vi "Complete Measurament RT.vi"() -> ()   [LabVIEW 2014]
uses:
  <vilib>/Platform/TimedLoop/XDataNode/timing_clust.ctl
  <vilib>/Platform/TimedLoop/XDataNode/nitl_modes.ctl
  <vilib>/Platform/TimedLoop/XDataNode/wakeup.ctl
  <vilib>/Analysis/3filter.llb/Filter Passband Type.ctl
  <vilib>/Analysis/Matrix/Datatypes/RealMatrix.ctl
  <vilib>/FPGAPlugInAG/sbRIO-9636/niLvFpga_Open_sbRIO-9636.vi
  <vilib>/rvi/interface/common/dynamic/niFpgaDynamicAddResources.vi
  <vilib>/FPGAPlugInAG/Dynamic/niLvFpga_Reset_Dynamic.vi
  <vilib>/Utility/error.llb/Error Cluster From Error Code.vi
  <vilib>/rvi/errors/niLvFpgaAdjustHostInterfaceError.vi
  <vilib>/rvi/interface/common/niFpgaWaitOnOcc.vi
  <vilib>/Analysis/3filter.llb/Butterworth Filter (DBL).vi
  <vilib>/FPGAPlugInAG/Dynamic/niLvFpga_Run_Dynamic.vi
  <vilib>/FPGAPlugInAG/Dynamic/niLvFpga_Abort_Dynamic.vi
  <vilib>/FPGAPlugInAG/Dynamic/niLvFpga_Close_Dynamic.vi
  <vilib>/rvi/interface/nirviOpenFPGA/nirviOpenFPGA.xnode
  FPGA Bitfiles/LaserDistanceSen_FPGATarget_N-ParametricDoub_YVLbjAYtdP4.lvbitx
  FPGA Target/Test VIs/N-Parametric Double FFT Mesurament Test.vi
  FPGA Bitfiles/LaserDistanceSen_FPGATarget_N-ParametricDoub_qx5IM88U9d4.lvbitx
  FPGA Target/Test VIs/N-Parametric Double FFT Mesurament Test SLOW.vi
  <vilib>/rvi/interface/nirviMethod/nirviMethod.xnode
  <vilib>/rvi/interface/nirviReadWriteControl/nirviReadWriteControl.xnode
  <vilib>/Platform/TimedLoop/XDataNode/XDataNode.xnode
  <vilib>/rvi/interface/nirviCloseFPGA/nirviCloseFPGA.xnode
  <vilib>/FPGAPlugInAG/Dynamic/niLvFpga_ConfigureFifo_Dynamic.vi
  <vilib>/rvi/errors/niLvFpgaMergeErrorWithErrorCode.vi
  <vilib>/FPGAPlugInAG/Dynamic/niLvFpga_StartFifo_Dynamic.vi
  <vilib>/rvi/interface/Simulation/niFpgaSimulationCallBeginRW.vi
  <vilib>/FPGAPlugInAG/Dynamic/niLvFpga_ReadFifo_Dynamic.vi
  <vilib>/Platform/TimedLoop/XDataNode/XDNodeRunTimeDep.lvlib
  NiFpgaLv.dll
  <vilib>/Analysis/NI_AALBase.lvlib
  <vilib>/Analysis/Matrix/NI_Matrix.lvlib
panel:
  out "Distance ONLINE":dbl[](graph)
  in  "Low cutoff freq":dbl=200000.0 format="%#_13g"
  in  "Tri Low pass filter":bool
  in  "3 point interpolation algorithm":bool
  in  "Mov mean":bool
  out "moving mean speed":dbl format="%0.7f"
  out "moving standard deviation rel speed":dbl format="%0.7f"
  in  "#movesignal 2":i32=100
  out "moving freq mean":dbl
  in  "Tab Control":enum32{"5 bin", "5 bin mean", "Distance "}(tab)=enum."Distance "
  out "5 bin FALL":T1(graph) caption="5 freq fall"
  out "5 bin RISE":T1(graph)
  out "5 bin mean/std FALL":T2(graph)
  in  "#meanBin":i32=100
  out "5 bin mean/std RISE":T2(graph)
  out "Distance and error":T1(graph)
  out "Speed and error":T1(graph)
  in  "Lin Mes":bool
  in  "step (m)":dbl=0.0001
  out "Max peak-peak error (m)":dbl
  out "Mean error (m)":dbl
  in  "Plot":bool
  in  "Sample /Modulation Frequency":enum32{"40MHz/32KHz", "30MHz/24Khz"}(radio)=enum."30MHz/24Khz"
  in  "#movesignal":i32=100
  out "moving standard deviation rel":dbl format="%0.7f"
  out "moving mean":dbl format="%0.7f"
  out "StdDev Rel 1":dbl
  out "StdDev Rel 2":dbl
  out "Warning":bool
  out "Velocity (m/s)":dbl
  out "Distance (m)":dbl
  out "Mean Frequency":dbl
  out "Rise array size":i32
  out "Fall array size":i32
  out "Mean Frequency Rising (Hz)":dbl
  out "Mean Frequency Falling (Hz)":dbl
  in  "tieni premuto per":i32=100
  in  "Triangular Multiply Factor":dbl[](array[numeric])=[1.0, 0.8, 0.95, 0.85, 0.9]
  out "RISING Second Edge N-FFT":dbl[](graph)
  in  "Enable triangular scaling":bool=TRUE
  in  "Triangolo dritto?":bool
  out "FALLING First Edge N-FFT":dbl[](graph)
  in  "#Signals":u32(slide)=5 scale=1.0..5.0
  in  "stop":bool
  in  "Initial Latency points":u32(slide) scale=0.0..1249.0
  out "Elements Remaining FFT":u32
  out "Elements Remaining Signal":u32
  out "N-Signals":dbl[](graph)
  in  "Snapshot":bool
  in  "Windowing":T3(ring)=enum."Hanning"
  in  "first bin":i32=5
  in  "last bin":i32=255
  in  "lower limit 2":u32(slide)=738 scale=625.0..738.0
  in  "lower limit 1":u32(slide)=113 scale=0.0..113.0
  # "OFFLINE parameters"
  # "200k/400k"
  # "Max Detection FFT bin range"
  # "WARNING:\nOnce pressed wait untill the end of operation"
  # "Distance"
  # "Mean"
  # "Velocity"
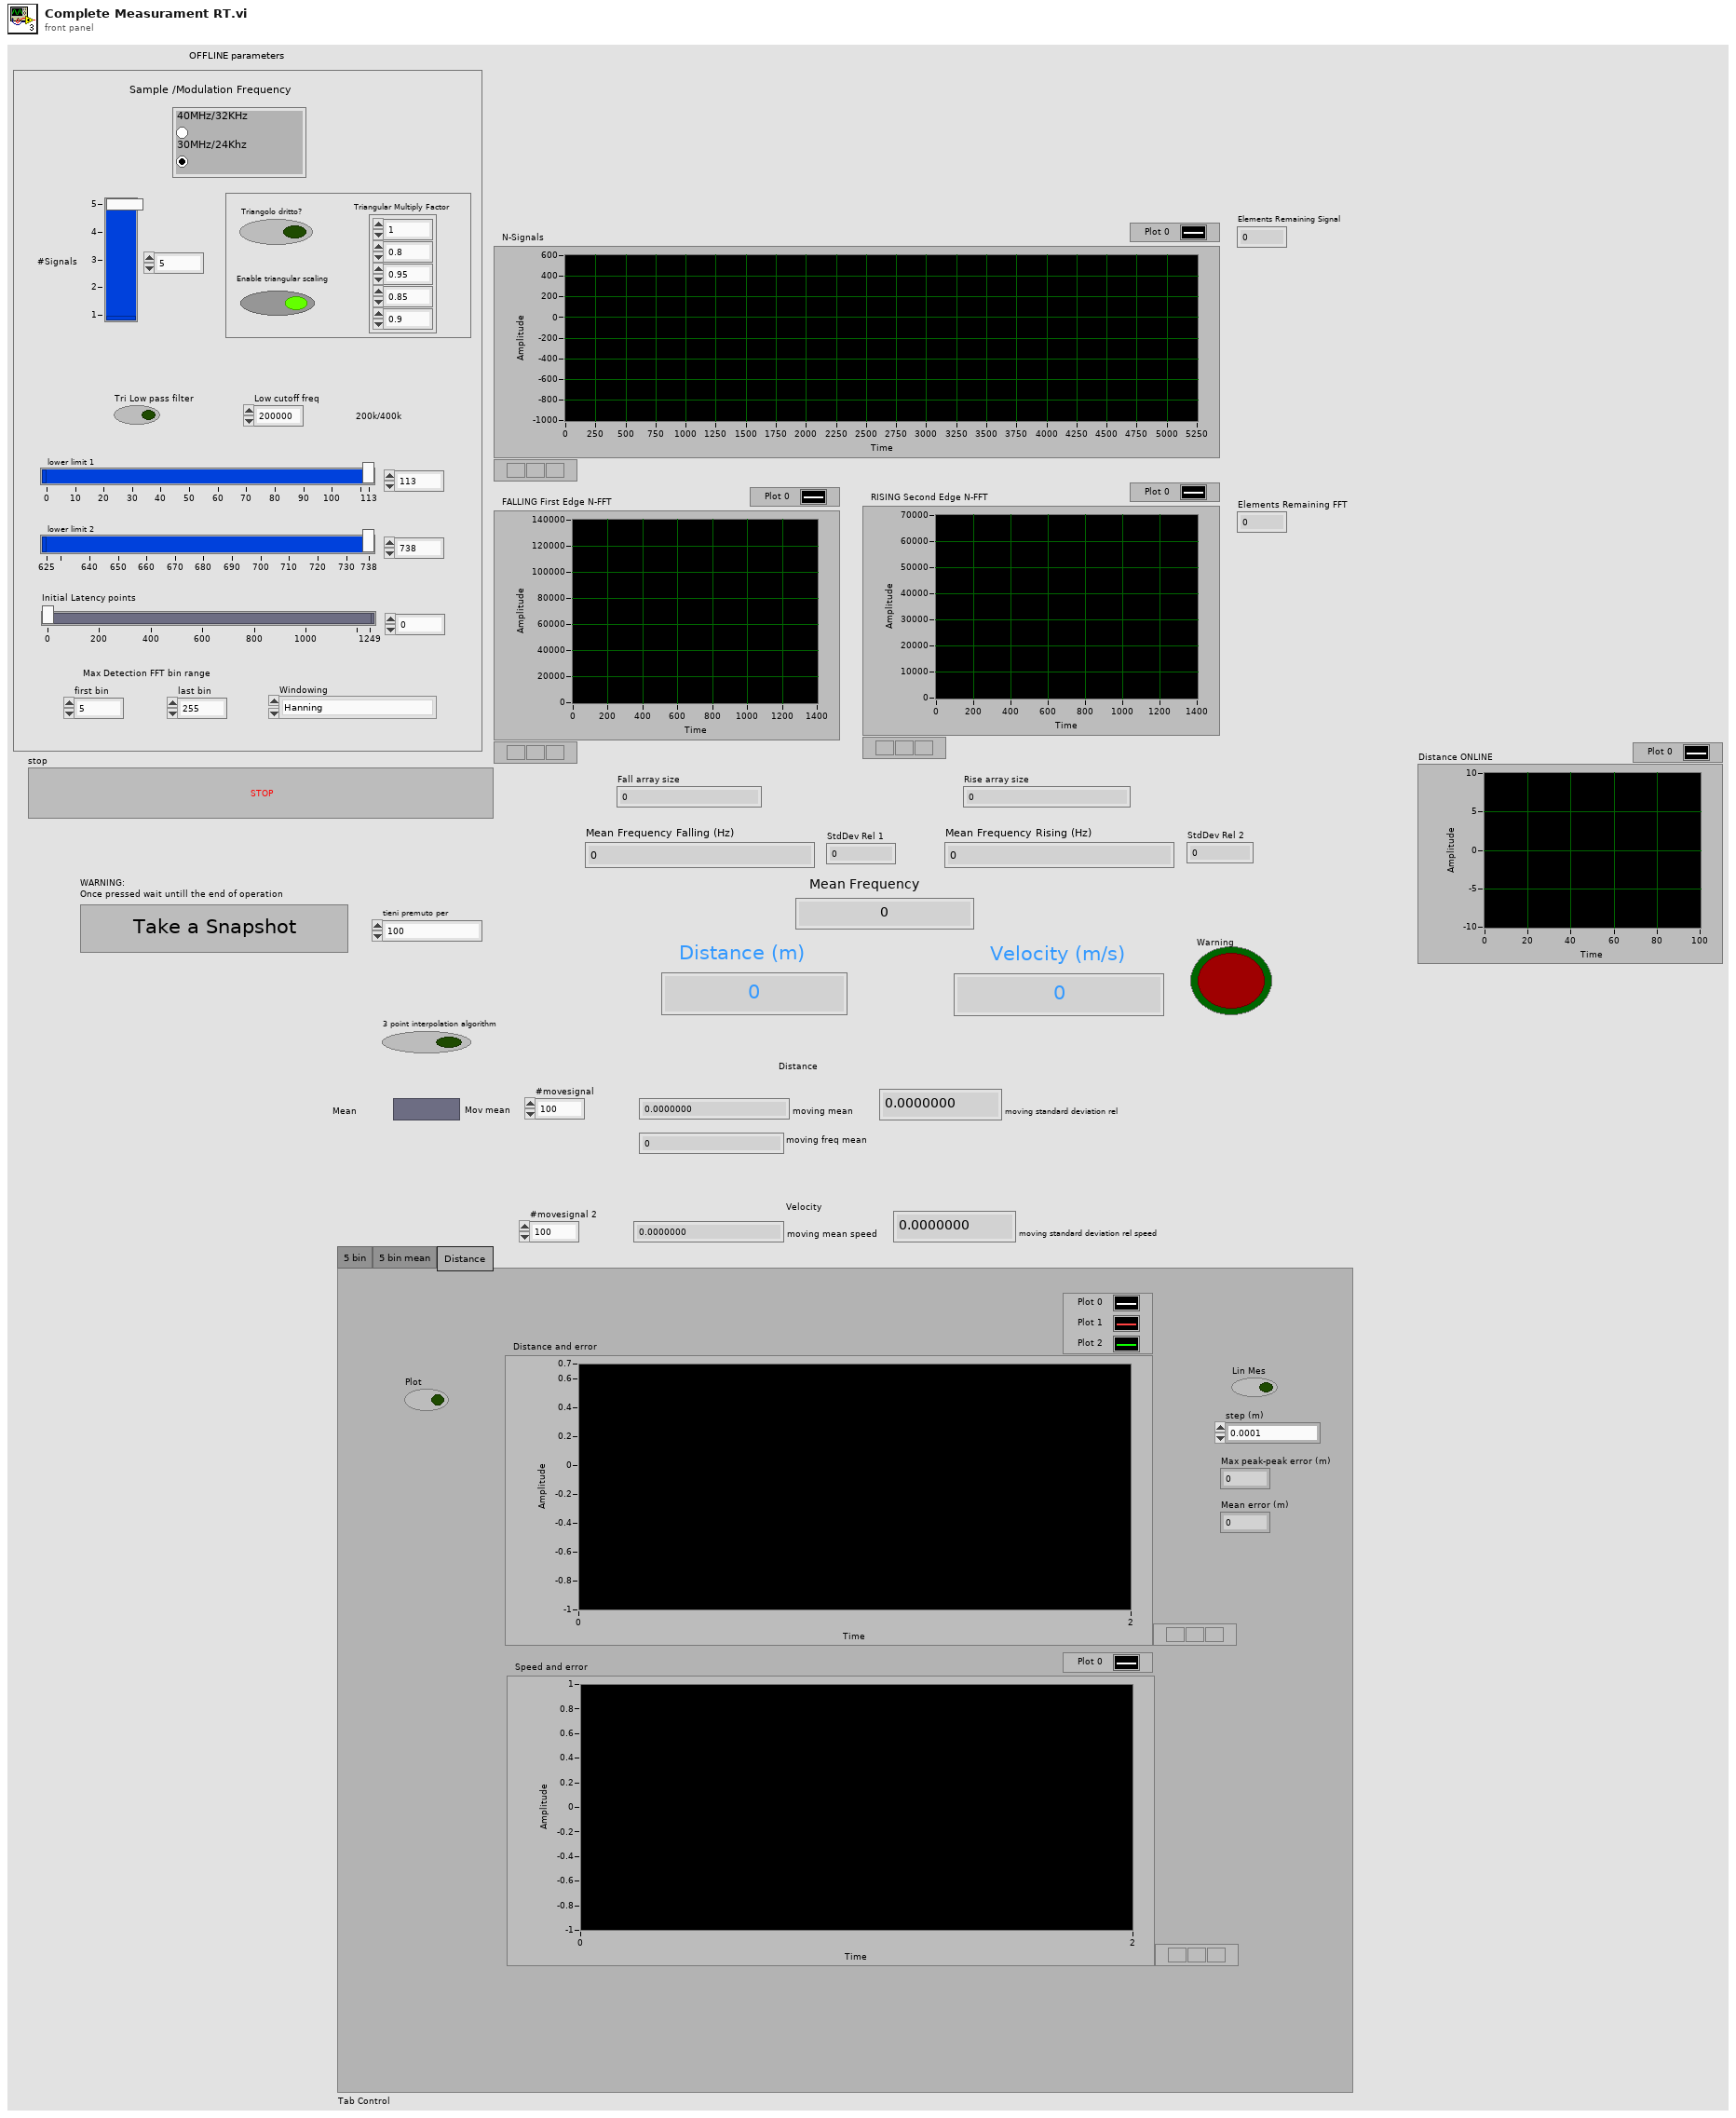
[diagram p1: front panel]
types:
  T1 = cluster{"[0]":dbl, "[1]":dbl, "[2]":dbl, "[3]":dbl, "[4]":dbl, "[5]":dbl, "[6]":dbl, "[7]":dbl, "[8]":dbl}
  T2 = cluster{"Array[0]":dbl, "Array[1]":dbl, "Array[2]":dbl, "Array[3]":dbl, "Array[4]":dbl, "Array[5]":dbl, "Array[6]":dbl, "Array[7]":dbl, "Array[8]":dbl}
  T3 = enum16{"None", "Hanning", "Hamming", "Blackman", "Blackman-Harris"}
  T4 = typedef "NI_AALBase.lvlib/Filter Passband Type.ctl" = enum32{"Lowpass", "Highpass", "Bandpass", "Bandstop"}
  T5 = typedef "XDNodeRunTimeDep.lvlib/timing_clust.ctl" = cluster{"Expected End [f-1]":u64, "Actual End [f-1]":u64, "Finished Late? [f-1]":bool, "Expected End [i-1]":u64, "Actual End [i-1]":u64, "Finished Late? [i-1]":bool, "Expected Start [i]":u64, "Actual Start [i]":u64, "Expected Start [f]":u64, "Actual Start [f]":u64, "Source Name":string, "Structure Name":string, "Period":i64, "Deadline":i64, "Offset":i64, "Start":i64, "Priority":i32, "Timeout":i32, "Mode":T6, "Wakeup Reason":T7, "Error":errorcluster, "Source Type":string, "Secondary Source Type":string, "Global End Time":u64, "Global Start Time":u64, "Frame Duration":u64, "Iteration Duration":u64, "Assigned CPU":i32, "I/O Scan Engine Mode":u32}
  T6 = typedef "XDNodeRunTimeDep.lvlib/nitl_modes.ctl" = enum32{"No Change", "Process missed periods, maintain original phase", "Discard missed periods, maintain original phase", "Process missed periods, ignore original phase", "Discard missed periods, ignore original phase"}
  T7 = typedef "XDNodeRunTimeDep.lvlib/wakeup.ctl" = enum32{"Normal", "Aborted", "Asynchronous wakeup", "Timing source error", "Timed loop error", "Timeout"}
  T8 = typedef "NI_Matrix.lvlib/RealMatrix.ctl" = dbl[][]
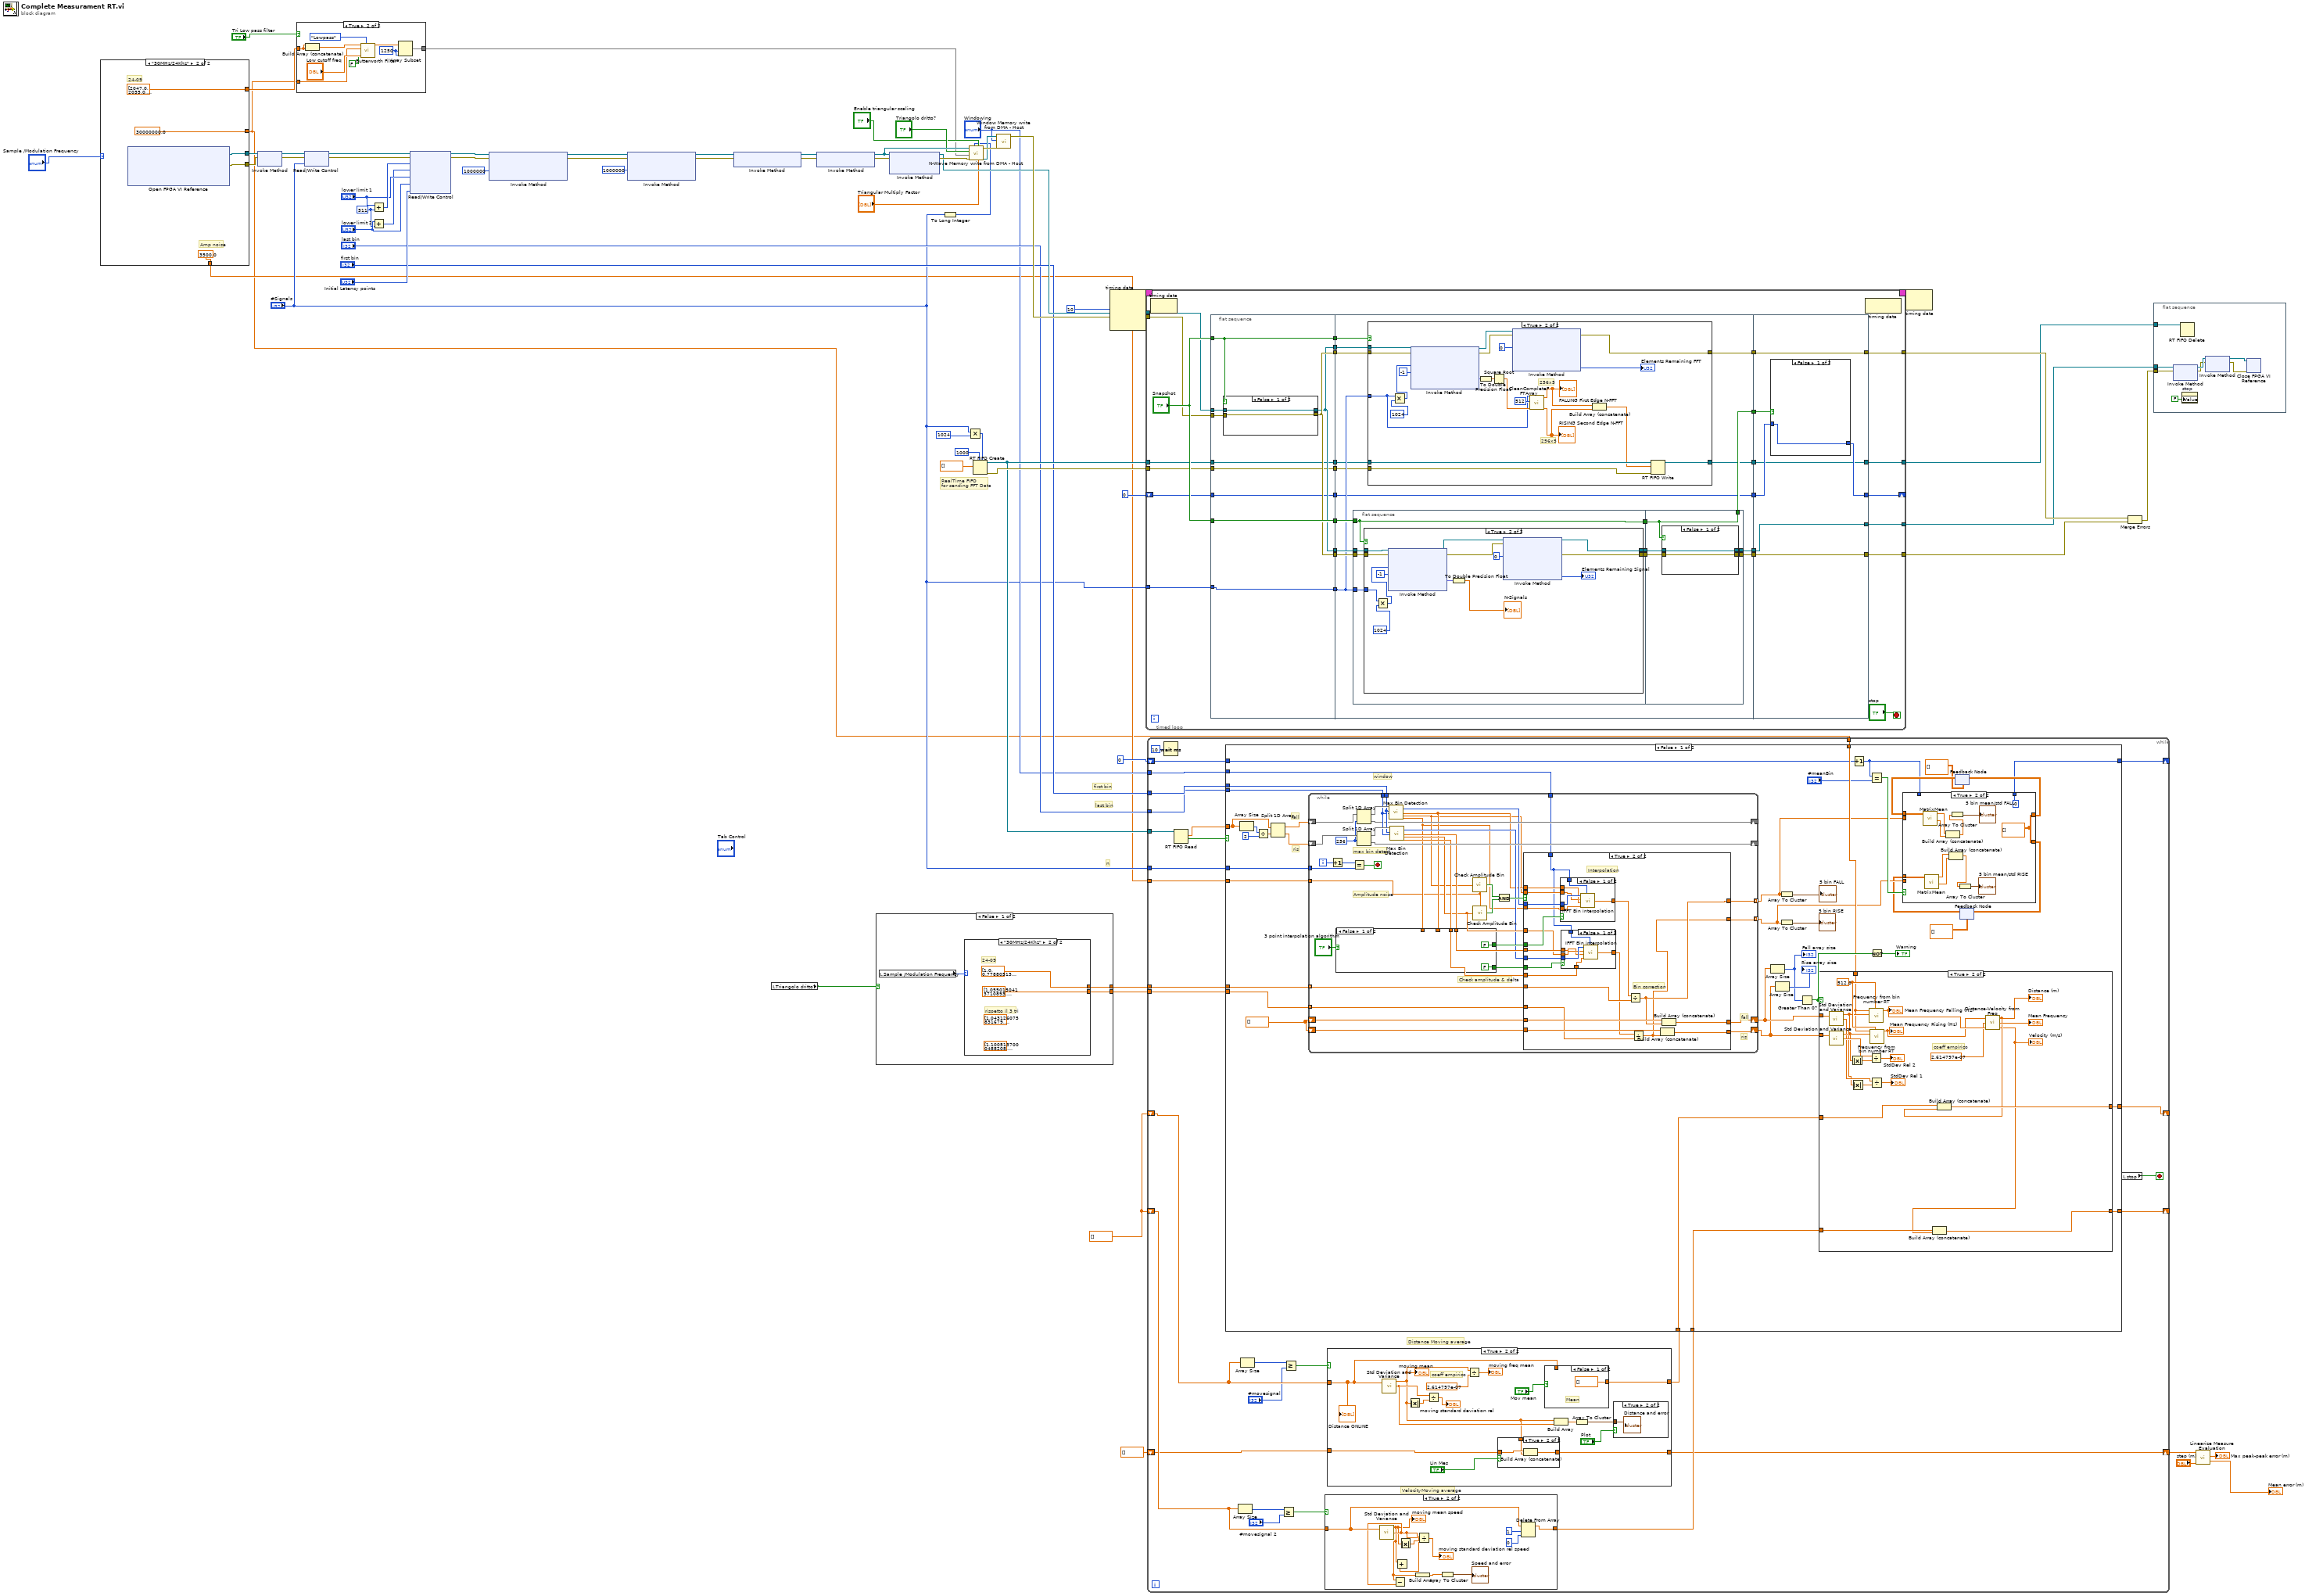
[diagram p0: block diagram]
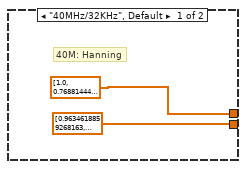
[diagram p3: hidden frame]
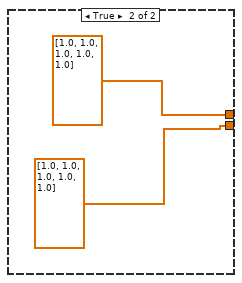
[diagram p4: hidden frame]
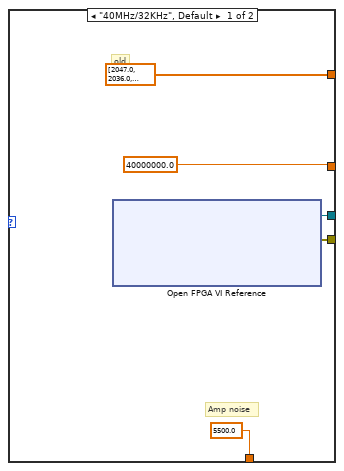
[diagram p5: hidden frame]
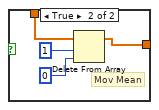
[diagram p10: hidden frame]
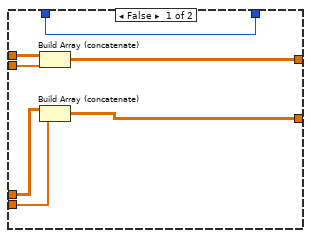
[diagram p11: hidden frame]
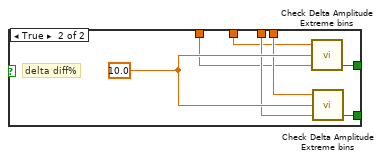
[diagram p13: hidden frame]
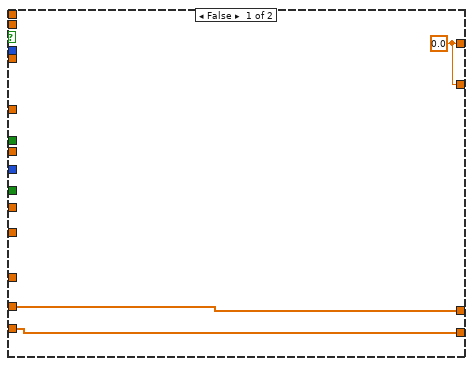
[diagram p14: hidden frame]
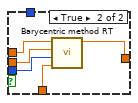
[diagram p15: hidden frame]
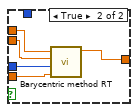
[diagram p16: hidden frame]
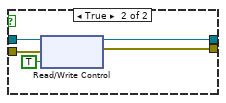
[diagram p18: hidden frame]
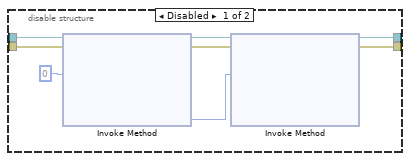
[diagram p20: hidden frame]
diagram:
  w11 = dbl[] [] ("appended array")
  w64 = u32 511 ("y")
  # "n"
  # "last bin"
  # "first bin"
  # "RealTime FIFO \nfor sending FFT Data"
  n1 = case shown="\"30MHz/24Khz\"" "Sample /Modulation Frequency" {
    tunnel: [w73 w78] -> w38
    tunnel: [w72 w77] -> w37
    tunnel: [40000000.0 30000000.0] -> w7
    tunnel: [5500.0 ("Threshold Amp") 3500.0 ("Threshold Amp")] -> w12
    tunnel: [dbl[] [2047.0, 2036.0, 2024.0, 2013.0, 2002.0, 1990.0, 1979.0, 1968.0, 1956.0, 1945.0, 1934.0, 1923.0, 1912.0, 1900.0, 1889.0, 1878.0, 1867.0, 1856.0, 1845.0, 1833.0, 1822.0, 1811.0, 1800.0, 1789.0, 1778.0, 1767.0, 1756.0, 1745.0, 1734.0, 1723.0, 1712.0, 1702.0, 1691.0, 1680.0, 1669.0, 1658.0, 1647.0, 1636.0, 1626.0, 1615.0, 1604.0, 1593.0, 1583.0, 1572.0, 1561.0, 1550.0, 1540.0, 1529.0, 1518.0, 1508.0, 1497.0, 1487.0, 1476.0, 1465.0, 1455.0, 1444.0, 1434.0, 1423.0, 1413.0, 1402.0, 1392.0, 1381.0, 1371.0, 1360.0, 1350.0, 1340.0, 1329.0, 1319.0, 1309.0, 1298.0, 1288.0, 1278.0, 1267.0, 1257.0, 1247.0, 1237.0, 1226.0, 1216.0, 1206.0, 1196.0, 1186.0, 1176.0, 1165.0, 1155.0, 1145.0, 1135.0, 1125.0, 1115.0, 1105.0, 1095.0, 1085.0, 1075.0, 1065.0, 1055.0, 1045.0, 1035.0, 1025.0, 1015.0, 1006.0, 996.0, 986.0, 976.0, 966.0, 956.0, 947.0, 937.0, 927.0, 917.0, 908.0, 898.0, 888.0, 879.0, 869.0, 859.0, 850.0, 837.0, 826.0, 816.0, 804.0, 796.0, 788.0, 778.0, 769.0, 758.0, 750.0, 743.0, 733.0, 724.0, 717.0, 709.0, 701.0, 693.0, 686.0, 677.0, 669.0, 661.0, 653.0, 645.0, 638.0, 630.0, 622.0, 615.0, 607.0, 599.0, 592.0, 583.0, 576.0, 569.0, 561.0, 554.0, 547.0, 539.0, 532.0, 525.0, 518.0, 509.0, 501.0, 492.0, 486.0, 478.0, 471.0, 463.0, 456.0, 450.0, 442.0, 435.0, 429.0, 421.0, 415.0, 408.0, 401.0, 394.0, 388.0, 381.0, 375.0, 368.0, 361.0, 355.0, 349.0, 342.0, 336.0, 330.0, 323.0, 317.0, 311.0, 304.0, 298.0, 292.0, 286.0, 279.0, 273.0, 267.0, 261.0, 255.0, 249.0, 242.0, 236.0, 230.0, 224.0, 218.0, 212.0, 206.0, 200.0, 194.0, 187.0, 181.0, 175.0, 169.0, 163.0, 157.0, 150.0, 144.0, 138.0, 132.0, 125.0, 119.0, 113.0, 107.0, 101.0, 95.0, 88.0, 82.0, 77.0, 71.0, 65.0, 59.0, 53.0, 47.0, 41.0, 35.0, 29.0, 23.0, 18.0, 11.0, 6.0, 0.0, -6.0, -12.0, -18.0, -23.0, -29.0, -35.0, -41.0, -47.0, -52.0, -58.0, -64.0, -69.0, -75.0, -81.0, -87.0, -92.0, -98.0, -104.0, -109.0, -115.0, -121.0, -126.0, -132.0, -138.0, -144.0, -149.0, -155.0, -161.0, -166.0, -172.0, -177.0, -183.0, -189.0, -194.0, -200.0, -205.0, -211.0, -216.0, -222.0, -227.0, -233.0, -238.0, -244.0, -249.0, -255.0, -260.0, -266.0, -271.0, -277.0, -283.0, -288.0, -294.0, -299.0, -304.0, -310.0, -315.0, -321.0, -326.0, -331.0, -337.0, -342.0, -348.0, -353.0, -358.0, -364.0, -369.0, -375.0, -380.0, -385.0, -391.0, -396.0, -402.0, -407.0, -413.0, -418.0, -423.0, -429.0, -434.0, -439.0, -445.0, -450.0, -456.0, -461.0, -466.0, -472.0, -477.0, -483.0, -488.0, -493.0, -499.0, -504.0, -510.0, -515.0, -520.0, -526.0, -531.0, -537.0, -542.0, -548.0, -553.0, -558.0, -564.0, -569.0, -574.0, -580.0, -585.0, -590.0, -596.0, -601.0, -606.0, -612.0, -617.0, -622.0, -628.0, -633.0, -638.0, -644.0, -649.0, -654.0, -660.0, -665.0, -670.0, -676.0, -681.0, -686.0, -692.0, -697.0, -702.0, -708.0, -713.0, -718.0, -723.0, -729.0, -734.0, -739.0, -744.0, -750.0, -755.0, -760.0, -765.0, -771.0, -776.0, -781.0, -786.0, -792.0, -797.0, -802.0, -807.0, -812.0, -818.0, -823.0, -828.0, -833.0, -839.0, -844.0, -849.0, -854.0, -859.0, -865.0, -870.0, -875.0, -880.0, -885.0, -891.0, -896.0, -901.0, -906.0, -911.0, -916.0, -922.0, -927.0, -932.0, -937.0, -943.0, -948.0, -953.0, -958.0, -963.0, -969.0, -974.0, -979.0, -984.0, -989.0, -995.0, -1000.0, -1005.0, -1010.0, -1015.0, -1021.0, -1026.0, -1031.0, -1036.0, -1041.0, -1047.0, -1052.0, -1057.0, -1062.0, -1067.0, -1073.0, -1078.0, -1083.0, -1088.0, -1093.0, -1099.0, -1104.0, -1109.0, -1114.0, -1119.0, -1124.0, -1130.0, -1135.0, -1140.0, -1145.0, -1150.0, -1156.0, -1161.0, -1166.0, -1171.0, -1176.0, -1182.0, -1187.0, -1192.0, -1197.0, -1202.0, -1207.0, -1213.0, -1218.0, -1223.0, -1228.0, -1233.0, -1238.0, -1244.0, -1249.0, -1254.0, -1259.0, -1264.0, -1269.0, -1275.0, -1280.0, -1285.0, -1290.0, -1295.0, -1300.0, -1305.0, -1311.0, -1316.0, -1321.0, -1326.0, -1331.0, -1336.0, -1342.0, -1347.0, -1352.0, -1357.0, -1362.0, -1367.0, -1372.0, -1378.0, -1383.0, -1388.0, -1393.0, -1398.0, -1403.0, -1408.0, -1414.0, -1419.0, -1424.0, -1429.0, -1434.0, -1439.0, -1444.0, -1450.0, -1455.0, -1460.0, -1465.0, -1470.0, -1475.0, -1480.0, -1486.0, -1491.0, -1496.0, -1501.0, -1506.0, -1511.0, -1516.0, -1522.0, -1527.0, -1532.0, -1537.0, -1542.0, -1547.0, -1552.0, -1558.0, -1563.0, -1568.0, -1573.0, -1578.0, -1583.0, -1588.0, -1593.0, -1599.0, -1604.0, -1609.0, -1614.0, -1619.0, -1624.0, -1629.0, -1634.0, -1640.0, -1645.0, -1650.0, -1655.0, -1660.0, -1665.0, -1670.0, -1675.0, -1681.0, -1686.0, -1691.0, -1696.0, -1701.0, -1706.0, -1711.0, -1716.0, -1722.0, -1727.0, -1732.0, -1737.0, -1742.0, -1747.0, -1752.0, -1757.0, -1762.0, -1768.0, -1773.0, -1778.0, -1783.0, -1788.0, -1793.0, -1798.0, -1803.0, -1808.0, -1814.0, -1819.0, -1824.0, -1829.0, -1834.0, -1839.0, -1844.0, -1849.0, -1854.0, -1859.0, -1865.0, -1870.0, -1875.0, -1880.0, -1885.0, -1890.0, -1895.0, -1900.0, -1905.0, -1911.0, -1916.0, -1921.0, -1926.0, -1931.0, -1936.0, -1941.0, -1946.0, -1951.0, -1956.0, -1961.0, -1967.0, -1972.0, -1977.0, -1982.0, -1987.0, -1992.0, -1997.0, -2002.0, -2007.0, -2012.0, -2017.0, -2023.0, -2028.0, -2033.0, -2038.0, -2043.0, -2048.0, -2047.0, -2034.0, -2021.0, -2009.0, -1996.0, -1983.0, -1970.0, -1957.0, -1945.0, -1932.0, -1919.0, -1907.0, -1894.0, -1881.0, -1869.0, -1856.0, -1844.0, -1831.0, -1819.0, -1806.0, -1794.0, -1781.0, -1769.0, -1757.0, -1744.0, -1732.0, -1719.0, -1707.0, -1695.0, -1682.0, -1670.0, -1658.0, -1646.0, -1634.0, -1621.0, -1609.0, -1597.0, -1585.0, -1573.0, -1561.0, -1549.0, -1537.0, -1525.0, -1513.0, -1501.0, -1489.0, -1477.0, -1465.0, -1453.0, -1441.0, -1429.0, -1417.0, -1405.0, -1394.0, -1382.0, -1370.0, -1358.0, -1347.0, -1335.0, -1323.0, -1312.0, -1300.0, -1288.0, -1277.0, -1265.0, -1254.0, -1242.0, -1231.0, -1219.0, -1208.0, -1196.0, -1185.0, -1173.0, -1162.0, -1150.0, -1139.0, -1128.0, -1116.0, -1105.0, -1094.0, -1083.0, -1071.0, -1060.0, -1049.0, -1038.0, -1027.0, -1015.0, -1004.0, -993.0, -982.0, -971.0, -960.0, -949.0, -938.0, -927.0, -916.0, -905.0, -894.0, -883.0, -873.0, -862.0, -851.0, -840.0, -829.0, -819.0, -808.0, -797.0, -786.0, -776.0, -765.0, -754.0, -744.0, -733.0, -722.0, -712.0, -697.0, -685.0, -674.0, -661.0, -652.0, -643.0, -632.0, -622.0, -610.0, -602.0, -594.0, -583.0, -574.0, -566.0, -558.0, -550.0, -542.0, -534.0, -525.0, -516.0, -507.0, -499.0, -491.0, -483.0, -475.0, -467.0, -459.0, -451.0, -443.0, -435.0, -426.0, -419.0, -411.0, -404.0, -396.0, -388.0, -381.0, -373.0, -366.0, -359.0, -349.0, -341.0, -331.0, -325.0, -317.0, -309.0, -301.0, -295.0, -288.0, -280.0, -273.0, -266.0, -259.0, -252.0, -246.0, -239.0, -231.0, -225.0, -219.0, -212.0, -205.0, -199.0, -192.0, -186.0, -180.0, -173.0, -167.0, -161.0, -155.0, -148.0, -142.0, -136.0, -130.0, -124.0, -118.0, -112.0, -106.0, -100.0, -94.0, -88.0, -82.0, -76.0, -70.0, -64.0, -58.0, -52.0, -46.0, -40.0, -34.0, -28.0, -21.0, -15.0, -9.0, -3.0, 2.0, 9.0, 15.0, 21.0, 27.0, 33.0, 39.0, 45.0, 51.0, 57.0, 63.0, 69.0, 75.0, 81.0, 86.0, 92.0, 98.0, 103.0, 110.0, 116.0, 121.0, 127.0, 133.0, 138.0, 144.0, 149.0, 155.0, 161.0, 166.0, 172.0, 177.0, 183.0, 189.0, 194.0, 200.0, 205.0, 211.0, 216.0, 221.0, 227.0, 232.0, 238.0, 243.0, 249.0, 254.0, 259.0, 265.0, 270.0, 276.0, 281.0, 286.0, 292.0, 297.0, 303.0, 308.0, 314.0, 319.0, 324.0, 329.0, 335.0, 340.0, 345.0, 351.0, 356.0, 361.0, 366.0, 371.0, 377.0, 382.0, 387.0, 392.0, 397.0, 403.0, 408.0, 413.0, 418.0, 423.0, 429.0, 434.0, 439.0, 444.0, 449.0, 454.0, 459.0, 464.0, 469.0, 474.0, 479.0, 484.0, 489.0, 494.0, 499.0, 504.0, 509.0, 514.0, 520.0, 525.0, 530.0, 535.0, 540.0, 545.0, 550.0, 555.0, 560.0, 565.0, 570.0, 575.0, 580.0, 585.0, 590.0, 595.0, 600.0, 605.0, 610.0, 615.0, 620.0, 625.0, 630.0, 636.0, 641.0, 646.0, 651.0, 656.0, 661.0, 666.0, 671.0, 676.0, 681.0, 686.0, 691.0, 696.0, 701.0, 706.0, 711.0, 716.0, 721.0, 726.0, 731.0, 736.0, 741.0, 746.0, 751.0, 756.0, 761.0, 765.0, 770.0, 775.0, 780.0, 785.0, 790.0, 795.0, 800.0, 805.0, 810.0, 815.0, 820.0, 825.0, 829.0, 834.0, 839.0, 844.0, 849.0, 854.0, 859.0, 864.0, 868.0, 873.0, 878.0, 883.0, 888.0, 893.0, 897.0, 902.0, 907.0, 912.0, 917.0, 921.0, 926.0, 931.0, 936.0, 941.0, 945.0, 950.0, 955.0, 960.0, 965.0, 969.0, 974.0, 979.0, 984.0, 988.0, 993.0, 998.0, 1003.0, 1007.0, 1012.0, 1017.0, 1022.0, 1027.0, 1031.0, 1036.0, 1041.0, 1046.0, 1051.0, 1055.0, 1060.0, 1065.0, 1070.0, 1075.0, 1079.0, 1084.0, 1089.0, 1094.0, 1098.0, 1103.0, 1108.0, 1113.0, 1118.0, 1122.0, 1127.0, 1132.0, 1137.0, 1141.0, 1146.0, 1151.0, 1156.0, 1161.0, 1165.0, 1170.0, 1175.0, 1180.0, 1184.0, 1189.0, 1194.0, 1199.0, 1204.0, 1208.0, 1213.0, 1218.0, 1223.0, 1227.0, 1232.0, 1237.0, 1242.0, 1246.0, 1251.0, 1256.0, 1261.0, 1265.0, 1270.0, 1275.0, 1280.0, 1284.0, 1289.0, 1294.0, 1299.0, 1303.0, 1308.0, 1313.0, 1318.0, 1322.0, 1327.0, 1332.0, 1336.0, 1341.0, 1346.0, 1351.0, 1355.0, 1360.0, 1365.0, 1370.0, 1374.0, 1379.0, 1384.0, 1388.0, 1393.0, 1398.0, 1403.0, 1407.0, 1412.0, 1417.0, 1421.0, 1426.0, 1431.0, 1436.0, 1440.0, 1445.0, 1450.0, 1454.0, 1459.0, 1464.0, 1469.0, 1473.0, 1478.0, 1483.0, 1487.0, 1492.0, 1497.0, 1502.0, 1506.0, 1511.0, 1516.0, 1520.0, 1525.0, 1530.0, 1535.0, 1539.0, 1544.0, 1549.0, 1553.0, 1558.0, 1563.0, 1567.0, 1572.0, 1577.0, 1582.0, 1586.0, 1591.0, 1596.0, 1600.0, 1605.0, 1610.0, 1614.0, 1619.0, 1624.0, 1628.0, 1633.0, 1638.0, 1643.0, 1647.0, 1652.0, 1657.0, 1661.0, 1666.0, 1671.0, 1675.0, 1680.0, 1685.0, 1689.0, 1694.0, 1699.0, 1703.0, 1708.0, 1713.0, 1717.0, 1722.0, 1727.0, 1731.0, 1736.0, 1741.0, 1746.0, 1750.0, 1755.0, 1760.0, 1764.0, 1769.0, 1774.0, 1778.0, 1783.0, 1788.0, 1792.0, 1797.0, 1802.0, 1806.0, 1811.0, 1816.0, 1820.0, 1825.0, 1830.0, 1834.0, 1839.0, 1844.0, 1848.0, 1853.0, 1858.0, 1862.0, 1867.0, 1871.0, 1876.0, 1881.0, 1885.0, 1890.0, 1895.0, 1899.0, 1904.0, 1909.0, 1913.0, 1918.0, 1923.0, 1927.0, 1932.0, 1937.0, 1941.0, 1946.0, 1951.0, 1955.0, 1960.0, 1965.0, 1969.0, 1974.0, 1978.0, 1983.0, 1988.0, 1992.0, 1997.0, 2002.0, 2006.0, 2011.0, 2016.0, 2020.0, 2025.0, 2029.0, 2034.0, 2039.0, 2043.0, 2048.0] ("Complete SkewTri") dbl[] [2047.0, 2035.0, 2022.0, 2010.0, 1997.0, 1985.0, 1972.0, 1960.0, 1948.0, 1935.0, 1923.0, 1911.0, 1899.0, 1886.0, 1874.0, 1862.0, 1850.0, 1838.0, 1825.0, 1813.0, 1801.0, 1789.0, 1777.0, 1765.0, 1753.0, 1741.0, 1729.0, 1717.0, 1705.0, 1693.0, 1681.0, 1669.0, 1657.0, 1645.0, 1634.0, 1622.0, 1610.0, 1598.0, 1586.0, 1575.0, 1563.0, 1551.0, 1540.0, 1528.0, 1516.0, 1505.0, 1493.0, 1481.0, 1470.0, 1458.0, 1447.0, 1435.0, 1424.0, 1412.0, 1401.0, 1389.0, 1378.0, 1366.0, 1355.0, 1344.0, 1332.0, 1321.0, 1310.0, 1298.0, 1287.0, 1276.0, 1265.0, 1253.0, 1242.0, 1231.0, 1220.0, 1209.0, 1198.0, 1186.0, 1175.0, 1164.0, 1153.0, 1142.0, 1131.0, 1120.0, 1109.0, 1098.0, 1087.0, 1076.0, 1065.0, 1055.0, 1044.0, 1033.0, 1022.0, 1011.0, 1000.0, 990.0, 979.0, 968.0, 958.0, 947.0, 936.0, 926.0, 915.0, 904.0, 894.0, 883.0, 873.0, 862.0, 852.0, 841.0, 831.0, 820.0, 810.0, 799.0, 789.0, 778.0, 768.0, 758.0, 747.0, 738.0, 727.0, 719.0, 712.0, 706.0, 700.0, 693.0, 687.0, 680.0, 674.0, 668.0, 661.0, 655.0, 648.0, 642.0, 636.0, 629.0, 623.0, 617.0, 610.0, 604.0, 598.0, 591.0, 584.0, 577.0, 569.0, 560.0, 552.0, 545.0, 538.0, 531.0, 525.0, 519.0, 512.0, 506.0, 500.0, 494.0, 488.0, 482.0, 476.0, 470.0, 464.0, 458.0, 452.0, 446.0, 436.0, 430.0, 424.0, 418.0, 412.0, 406.0, 400.0, 394.0, 388.0, 382.0, 376.0, 370.0, 364.0, 358.0, 352.0, 346.0, 338.0, 332.0, 325.0, 319.0, 313.0, 307.0, 301.0, 295.0, 290.0, 284.0, 278.0, 272.0, 267.0, 261.0, 255.0, 249.0, 244.0, 238.0, 232.0, 227.0, 221.0, 215.0, 209.0, 204.0, 198.0, 192.0, 187.0, 181.0, 175.0, 170.0, 164.0, 158.0, 153.0, 147.0, 141.0, 136.0, 130.0, 124.0, 119.0, 113.0, 108.0, 102.0, 96.0, 91.0, 85.0, 79.0, 74.0, 68.0, 62.0, 57.0, 51.0, 45.0, 39.0, 34.0, 28.0, 22.0, 16.0, 11.0, 5.0, 0.0, -6.0, -11.0, -17.0, -22.0, -28.0, -33.0, -39.0, -44.0, -50.0, -55.0, -61.0, -66.0, -72.0, -77.0, -83.0, -88.0, -94.0, -99.0, -105.0, -110.0, -116.0, -121.0, -127.0, -132.0, -137.0, -143.0, -148.0, -154.0, -159.0, -165.0, -170.0, -176.0, -181.0, -186.0, -192.0, -197.0, -203.0, -208.0, -214.0, -219.0, -224.0, -230.0, -235.0, -241.0, -246.0, -251.0, -257.0, -262.0, -268.0, -273.0, -278.0, -284.0, -289.0, -295.0, -300.0, -305.0, -311.0, -316.0, -321.0, -327.0, -332.0, -337.0, -343.0, -348.0, -354.0, -359.0, -364.0, -370.0, -375.0, -380.0, -386.0, -391.0, -397.0, -402.0, -407.0, -413.0, -418.0, -423.0, -429.0, -434.0, -439.0, -445.0, -450.0, -455.0, -461.0, -466.0, -471.0, -477.0, -482.0, -487.0, -493.0, -498.0, -503.0, -509.0, -514.0, -519.0, -525.0, -530.0, -535.0, -540.0, -546.0, -551.0, -556.0, -562.0, -567.0, -572.0, -578.0, -583.0, -588.0, -593.0, -599.0, -604.0, -609.0, -615.0, -620.0, -625.0, -630.0, -636.0, -641.0, -646.0, -651.0, -657.0, -662.0, -667.0, -673.0, -678.0, -683.0, -688.0, -694.0, -699.0, -704.0, -709.0, -715.0, -720.0, -725.0, -730.0, -736.0, -741.0, -746.0, -751.0, -757.0, -762.0, -767.0, -772.0, -778.0, -783.0, -788.0, -793.0, -799.0, -804.0, -809.0, -814.0, -820.0, -825.0, -830.0, -835.0, -841.0, -846.0, -851.0, -856.0, -862.0, -867.0, -872.0, -877.0, -883.0, -888.0, -893.0, -898.0, -903.0, -909.0, -914.0, -919.0, -924.0, -930.0, -935.0, -940.0, -945.0, -951.0, -956.0, -961.0, -966.0, -971.0, -977.0, -982.0, -987.0, -992.0, -998.0, -1003.0, -1008.0, -1013.0, -1018.0, -1024.0, -1029.0, -1034.0, -1039.0, -1045.0, -1050.0, -1055.0, -1060.0, -1065.0, -1071.0, -1076.0, -1081.0, -1086.0, -1092.0, -1097.0, -1102.0, -1107.0, -1112.0, -1118.0, -1123.0, -1128.0, -1133.0, -1138.0, -1144.0, -1149.0, -1154.0, -1159.0, -1165.0, -1170.0, -1175.0, -1180.0, -1185.0, -1191.0, -1196.0, -1201.0, -1206.0, -1211.0, -1217.0, -1222.0, -1227.0, -1232.0, -1237.0, -1243.0, -1248.0, -1253.0, -1258.0, -1263.0, -1269.0, -1274.0, -1279.0, -1284.0, -1289.0, -1295.0, -1300.0, -1305.0, -1310.0, -1315.0, -1321.0, -1326.0, -1331.0, -1336.0, -1341.0, -1347.0, -1352.0, -1357.0, -1362.0, -1367.0, -1373.0, -1378.0, -1383.0, -1388.0, -1393.0, -1399.0, -1404.0, -1409.0, -1414.0, -1419.0, -1425.0, -1430.0, -1435.0, -1440.0, -1445.0, -1450.0, -1456.0, -1461.0, -1466.0, -1471.0, -1476.0, -1482.0, -1487.0, -1492.0, -1497.0, -1502.0, -1508.0, -1513.0, -1518.0, -1523.0, -1528.0, -1534.0, -1539.0, -1544.0, -1549.0, -1554.0, -1560.0, -1565.0, -1570.0, -1575.0, -1580.0, -1586.0, -1591.0, -1596.0, -1601.0, -1606.0, -1612.0, -1617.0, -1622.0, -1627.0, -1632.0, -1637.0, -1643.0, -1648.0, -1653.0, -1658.0, -1663.0, -1669.0, -1674.0, -1679.0, -1684.0, -1689.0, -1695.0, -1700.0, -1705.0, -1710.0, -1715.0, -1721.0, -1726.0, -1731.0, -1736.0, -1741.0, -1747.0, -1752.0, -1757.0, -1762.0, -1767.0, -1773.0, -1778.0, -1783.0, -1788.0, -1793.0, -1799.0, -1804.0, -1809.0, -1814.0, -1819.0, -1825.0, -1830.0, -1835.0, -1840.0, -1845.0, -1851.0, -1856.0, -1861.0, -1866.0, -1871.0, -1876.0, -1882.0, -1887.0, -1892.0, -1897.0, -1902.0, -1908.0, -1913.0, -1918.0, -1923.0, -1928.0, -1934.0, -1939.0, -1944.0, -1949.0, -1954.0, -1960.0, -1965.0, -1970.0, -1975.0, -1980.0, -1986.0, -1991.0, -1996.0, -2001.0, -2006.0, -2012.0, -2017.0, -2022.0, -2027.0, -2032.0, -2038.0, -2043.0, -2048.0, -2047.0, -2037.0, -2027.0, -2017.0, -2007.0, -1997.0, -1987.0, -1977.0, -1967.0, -1957.0, -1947.0, -1937.0, -1927.0, -1917.0, -1907.0, -1897.0, -1888.0, -1878.0, -1868.0, -1858.0, -1848.0, -1838.0, -1828.0, -1819.0, -1809.0, -1799.0, -1789.0, -1780.0, -1770.0, -1760.0, -1750.0, -1741.0, -1731.0, -1721.0, -1712.0, -1702.0, -1692.0, -1683.0, -1673.0, -1663.0, -1654.0, -1644.0, -1635.0, -1625.0, -1615.0, -1606.0, -1596.0, -1587.0, -1577.0, -1568.0, -1558.0, -1549.0, -1539.0, -1530.0, -1520.0, -1511.0, -1501.0, -1492.0, -1483.0, -1473.0, -1464.0, -1454.0, -1445.0, -1436.0, -1426.0, -1417.0, -1408.0, -1398.0, -1389.0, -1380.0, -1371.0, -1361.0, -1352.0, -1343.0, -1334.0, -1324.0, -1315.0, -1306.0, -1297.0, -1288.0, -1278.0, -1269.0, -1260.0, -1251.0, -1242.0, -1233.0, -1224.0, -1215.0, -1205.0, -1196.0, -1187.0, -1178.0, -1169.0, -1160.0, -1151.0, -1142.0, -1133.0, -1124.0, -1115.0, -1106.0, -1097.0, -1088.0, -1080.0, -1071.0, -1062.0, -1053.0, -1044.0, -1035.0, -1026.0, -1017.0, -1009.0, -1000.0, -991.0, -982.0, -973.0, -965.0, -953.0, -944.0, -935.0, -920.0, -906.0, -889.0, -871.0, -854.0, -842.0, -834.0, -826.0, -818.0, -810.0, -802.0, -794.0, -786.0, -778.0, -770.0, -762.0, -754.0, -746.0, -739.0, -731.0, -723.0, -715.0, -707.0, -699.0, -690.0, -682.0, -672.0, -661.0, -651.0, -639.0, -627.0, -616.0, -606.0, -598.0, -591.0, -584.0, -577.0, -570.0, -563.0, -556.0, -549.0, -542.0, -535.0, -528.0, -520.0, -513.0, -506.0, -499.0, -492.0, -485.0, -478.0, -471.0, -464.0, -457.0, -451.0, -444.0, -437.0, -430.0, -423.0, -416.0, -409.0, -400.0, -390.0, -382.0, -373.0, -364.0, -356.0, -349.0, -343.0, -336.0, -330.0, -323.0, -317.0, -310.0, -304.0, -297.0, -291.0, -284.0, -278.0, -271.0, -265.0, -258.0, -252.0, -245.0, -239.0, -232.0, -226.0, -219.0, -213.0, -207.0, -200.0, -194.0, -187.0, -181.0, -175.0, -168.0, -162.0, -156.0, -149.0, -143.0, -136.0, -128.0, -121.0, -114.0, -107.0, -100.0, -93.0, -87.0, -80.0, -74.0, -68.0, -62.0, -56.0, -50.0, -44.0, -38.0, -32.0, -26.0, -20.0, -14.0, -8.0, -2.0, 5.0, 11.0, 17.0, 23.0, 29.0, 35.0, 41.0, 47.0, 53.0, 59.0, 65.0, 70.0, 76.0, 82.0, 88.0, 94.0, 100.0, 106.0, 112.0, 118.0, 124.0, 130.0, 136.0, 142.0, 148.0, 154.0, 161.0, 167.0, 174.0, 180.0, 186.0, 192.0, 198.0, 204.0, 210.0, 215.0, 221.0, 227.0, 233.0, 238.0, 244.0, 250.0, 255.0, 261.0, 267.0, 273.0, 278.0, 284.0, 290.0, 295.0, 301.0, 307.0, 312.0, 318.0, 324.0, 329.0, 335.0, 341.0, 346.0, 352.0, 358.0, 363.0, 369.0, 374.0, 380.0, 386.0, 391.0, 397.0, 402.0, 408.0, 414.0, 419.0, 425.0, 430.0, 436.0, 441.0, 447.0, 453.0, 458.0, 464.0, 470.0, 475.0, 481.0, 487.0, 493.0, 499.0, 504.0, 510.0, 516.0, 521.0, 527.0, 532.0, 538.0, 543.0, 549.0, 554.0, 560.0, 565.0, 571.0, 576.0, 582.0, 587.0, 593.0, 598.0, 604.0, 609.0, 614.0, 620.0, 625.0, 631.0, 636.0, 642.0, 647.0, 653.0, 658.0, 663.0, 669.0, 674.0, 680.0, 685.0, 691.0, 696.0, 701.0, 707.0, 712.0, 718.0, 723.0, 728.0, 734.0, 739.0, 745.0, 750.0, 755.0, 761.0, 766.0, 772.0, 777.0, 782.0, 788.0, 793.0, 798.0, 804.0, 809.0, 815.0, 820.0, 826.0, 831.0, 837.0, 842.0, 847.0, 853.0, 858.0, 863.0, 869.0, 874.0, 880.0, 885.0, 890.0, 895.0, 901.0, 906.0, 911.0, 917.0, 922.0, 927.0, 933.0, 938.0, 943.0, 948.0, 954.0, 959.0, 964.0, 970.0, 975.0, 980.0, 985.0, 991.0, 996.0, 1001.0, 1006.0, 1012.0, 1017.0, 1022.0, 1027.0, 1033.0, 1038.0, 1043.0, 1048.0, 1054.0, 1059.0, 1064.0, 1069.0, 1075.0, 1080.0, 1085.0, 1090.0, 1096.0, 1101.0, 1106.0, 1111.0, 1116.0, 1122.0, 1127.0, 1132.0, 1137.0, 1143.0, 1148.0, 1153.0, 1158.0, 1163.0, 1169.0, 1174.0, 1179.0, 1184.0, 1190.0, 1195.0, 1200.0, 1205.0, 1211.0, 1216.0, 1221.0, 1226.0, 1231.0, 1237.0, 1242.0, 1247.0, 1252.0, 1257.0, 1262.0, 1268.0, 1273.0, 1278.0, 1283.0, 1288.0, 1293.0, 1298.0, 1304.0, 1309.0, 1314.0, 1319.0, 1324.0, 1329.0, 1334.0, 1340.0, 1345.0, 1350.0, 1355.0, 1360.0, 1365.0, 1370.0, 1375.0, 1381.0, 1386.0, 1391.0, 1396.0, 1401.0, 1406.0, 1411.0, 1416.0, 1421.0, 1427.0, 1432.0, 1437.0, 1442.0, 1447.0, 1452.0, 1457.0, 1462.0, 1467.0, 1472.0, 1478.0, 1483.0, 1488.0, 1493.0, 1498.0, 1503.0, 1508.0, 1513.0, 1518.0, 1523.0, 1528.0, 1534.0, 1539.0, 1544.0, 1549.0, 1554.0, 1559.0, 1564.0, 1569.0, 1574.0, 1579.0, 1584.0, 1589.0, 1595.0, 1600.0, 1605.0, 1610.0, 1615.0, 1620.0, 1625.0, 1630.0, 1635.0, 1640.0, 1645.0, 1650.0, 1655.0, 1660.0, 1666.0, 1671.0, 1676.0, 1681.0, 1686.0, 1691.0, 1696.0, 1701.0, 1706.0, 1711.0, 1716.0, 1721.0, 1726.0, 1731.0, 1736.0, 1741.0, 1746.0, 1751.0, 1757.0, 1762.0, 1767.0, 1772.0, 1777.0, 1782.0, 1787.0, 1792.0, 1797.0, 1802.0, 1807.0, 1812.0, 1817.0, 1822.0, 1827.0, 1832.0, 1837.0, 1842.0, 1847.0, 1852.0, 1857.0, 1862.0, 1867.0, 1872.0, 1877.0, 1883.0, 1888.0, 1893.0, 1898.0, 1903.0, 1908.0, 1913.0, 1918.0, 1923.0, 1928.0, 1933.0, 1938.0, 1943.0, 1948.0, 1953.0, 1958.0, 1963.0, 1968.0, 1973.0, 1978.0, 1983.0, 1988.0, 1993.0, 1998.0, 2003.0, 2008.0, 2013.0, 2018.0, 2023.0, 2028.0, 2033.0, 2038.0, 2043.0, 2048.0] ("appended array")] -> w9
    frame "40MHz/32KHz", Default {
      # "old"
      # "Amp noise"
      n2 = xnode "Open FPGA VI Reference"() -> ("FPGA VI Reference Out"=w73:refnum<k20>, "error out"=w72:errorcluster)  [unwired: 2 in]
    }
    frame "30MHz/24Khz" {
      # "24-09"
      # "Amp noise"
      n3 = xnode "Open FPGA VI Reference"() -> ("FPGA VI Reference Out"=w78:refnum<k20>, "error out"=w77:errorcluster)  [unwired: 2 in]
    }
  }
  n4 = xnode "Invoke Method"("FPGA VI Reference In"=w38, "error in"=w37) -> ("FPGA VI Reference Out"=w35:refnum<k20>, "error out"=w36:errorcluster)
  n5 = case shown="True" "Tri Low pass filter" {
    tunnel: w9 -> [w79 w84]
    tunnel: [w79 w80] -> w8
    tunnel: w7 -> [_ w85]
    frame False {
    }
    frame True {
      w81 = 1250 ("length")
      n6 = Build Array (concatenate)(w84, w84) -> (w83:dbl[])
      n7 = call-poly <vilib>:"Butterworth Filter.vi"("init/cont (init:F)"=FALSE, "filter type"=Filter_Passband_Type."Lowpass", "low cutoff freq: fl"="Low cutoff freq", "sampling freq: fs"=w85, "X"=w83) -> ("Filtered X"=w82:dbl[])  [unwired: 3 in, 1 out]
      n8 = Array Subset(array=w82, index=w81, length=w81) -> (w80:dbl[])
    }
  }
  n9 = xnode "Read/Write Control"("FPGA VI Reference In"=w35, "error in"=w36, "n"="#Signals") -> ("FPGA VI Reference Out"=w34:refnum<k20>, "error out"=w33:errorcluster)
  n10 = Add(x="lower limit 1", y=w64) -> (x+y=w68:u32)
  n11 = Add(x="lower limit 2", y=w64) -> (x+y=w66:u32)
  n12 = xnode "Read/Write Control"("FPGA VI Reference In"=w34, "error in"=w33, "upper limit 1"=w68, "upper limit 2"=w66, "lower limit 1"="lower limit 1", "lower limit 2"="lower limit 2", "Latency points"="Initial Latency points") -> ("FPGA VI Reference Out"=w62:refnum<k20>, "error out"=w61:errorcluster)
  n13 = xnode "Invoke Method"("FPGA VI Reference In"=w62, "error in"=w61, "Requested Depth"=u32 1000000) -> ("FPGA VI Reference Out"=w49:refnum<k20>, "error out"=w50:errorcluster)  [unwired: 1 out]
  n14 = xnode "Invoke Method"("FPGA VI Reference In"=w49, "error in"=w50, "Requested Depth"=u32 1000000) -> ("FPGA VI Reference Out"=w56:refnum<k20>, "error out"=w57:errorcluster)  [unwired: 1 out]
  n15 = xnode "Invoke Method"("FPGA VI Reference In"=w56, "error in"=w57) -> ("FPGA VI Reference Out"=w47:refnum<k20>, "error out"=w48:errorcluster)
  n16 = local read "Triangolo dritto?"() -> (w10:bool)
  n17 = xnode "Invoke Method"("FPGA VI Reference In"=w47, "error in"=w48) -> ("FPGA VI Reference Out"=w42:refnum<k20>, "error out"=w55:errorcluster)
  n18 = case shown="False" w10 {
    tunnel: [w91 dbl[] [1.0, 1.0, 1.0, 1.0, 1.0] ("mean factor 1")] -> w15
    tunnel: [w90 dbl[] [1.0, 1.0, 1.0, 1.0, 1.0] ("mean factor 1")] -> w14
    frame False {
      n19 = local read "Sample /Modulation Frequency"() -> (w89:enum32{"40MHz/32KHz", "30MHz/24Khz"})
      n20 = case shown="\"30MHz/24Khz\"" w89 {
        tunnel: [dbl[] [1.0, 0.7688144425878637, 0.960709657195022, 0.8322860112544478, 0.9000054001812109] ("mean factor 1") dbl[] [1.0, 0.7788051374952276, 0.9586568902543302, 0.8395566206470091, 0.903068410955916] ("mean factor 1")] -> w91
        tunnel: [dbl[] [0.9634618859268163, 0.8014672128927146, 0.9212223217673626, 0.8422741314179902, 0.8798034158007506] ("mean factor 2") dbl[] [1.0550150413710893, 0.8807744280543515, 1.0096480344577006, 0.9233799836458207, 0.9653106595082892] ("mean factor 2")] -> w90
        frame "40MHz/32KHz", Default {
          # "40M: Hanning"
        }
        frame "30MHz/24Khz" {
          (unwired) dbl[] [1.1005137000488208, 0.9187587728292271, 1.053190192155029, 0.9632017388419849, 1.0069407202113718] ("x/y 2")
          (unwired) dbl[] [1.043126075831679, 0.812391946912948, 1.0, 0.8757634031340201, 0.9420142077279946] ("x/y")
          # "rispetto il 3 tri"
          # "24-09"
        }
      }
    }
    frame True {
    }
  }
  n21 = xnode "Invoke Method"("FPGA VI Reference In"=w42, "error in"=w55) -> ("FPGA VI Reference Out"=w43:refnum<k20>, "error out"=w46:errorcluster)  [unwired: 1 in]
  n22 = To Long Integer(number="#Signals") -> (32bit integer=w29:i32)
  n23 = Multiply(x="#Signals", y=u32 1024 ("elements in array (1)")) -> (x*y=w25:u32)
  n24 = call "N-Wave Memory write from DMA - Host.vi"("Triangular Multiply Factor"="Triangular Multiply Factor", "Enable triangular scaling"="Enable triangular scaling", "n"=w29, "error in"=w46, "Custom Triangular Signal (fal-ris)"=w8, "Triangolo dritto?"="Triangolo dritto?", "FPGA VI Reference In"=w42) -> ("FPGA VI Reference Out"=w44:refnum<k20>, "error out"=w45:errorcluster)  [unwired: 2 in, 1 out]
  n25 = RT FIFO Create(1:dbl[] [] ("double precision float"), 4:u32 1000 ("size (10)"), 6:w25) -> (8:w22:refnum<k33>, 11:w23:errorcluster)  [unwired: 5 in, 1 out]
  n26 = call "Window Memory write from DMA - Host.vi"("error in"=w45, "Enum"="Windowing", "FPGA VI Reference In"=w44) -> ("error out"=w63:errorcluster)  [unwired: 5 in, 3 out]
  n27 = node-c288(i64 10 ("Period")) -> (w41:T5)  [unwired: 3 in]
  n28 = timed-loop {
    tunnel: w43 -> [w122]
    tunnel: w63 -> [w123]
    tunnel: [w125] -> w54
    tunnel: [w126] -> w53
    tunnel: [w111] -> w51
    tunnel: "#Signals" -> [w108]
    timing: w41 -> [_]
    timing-out: [_] -> w40
    shift-right: [w104] -> _
    shift-left: 0 -> [w107]
    tunnel: w22 -> [w103]
    tunnel: w23 -> [w100]
    tunnel: [w98] -> w17
    stop <- "stop" stop-if-true
    n29 = node-c288() -> ()  [unwired: 1 in, 1 out]
    n30 = flat-sequence {
      tunnel: w122 -> [w135]
      tunnel: w123 -> [w136]
      tunnel: "Snapshot" -> [w133]
      tunnel: "Snapshot" -> [w138]
      tunnel: [w137] -> w121
      tunnel: [w138] -> w120
      tunnel: [w133] -> w119
      tunnel: [w137] -> w118
      tunnel: [w134] -> w117
      tunnel: [w134] -> w116
      tunnel: [w132] -> w109
      tunnel: w108 -> [w132]
      tunnel: w107 -> [w131]
      tunnel: [w131] -> w106
      tunnel: w103 -> [w130]
      tunnel: [w130] -> w102
      tunnel: [w129] -> w101
      tunnel: w100 -> [w129]
      tunnel: w121 -> [w159]
      tunnel: w120 -> [w153]
      tunnel: w119 -> [w156]
      tunnel: w118 -> [w155]
      tunnel: w117 -> [w154]
      tunnel: w116 -> [w160]
      tunnel: [w158] -> w115
      tunnel: [w157] -> w114
      tunnel: [w152] -> w113
      tunnel: [w151] -> w110
      tunnel: w109 -> [w150]
      tunnel: w106 -> [w149]
      tunnel: [w149] -> w105
      tunnel: w102 -> [w148]
      tunnel: w101 -> [w147]
      tunnel: [w146] -> w99
      tunnel: [w248] -> w125
      tunnel: [w249] -> w126
      tunnel: w115 -> [w249]
      tunnel: w114 -> [w248]
      tunnel: w113 -> [w246]
      tunnel: [w247] -> w111
      tunnel: w110 -> [w247]
      tunnel: w105 -> [w245]
      tunnel: [w244] -> w104
      tunnel: w99 -> [w243]
      tunnel: [w243] -> w98
      frame #0 {
        n31 = case shown="False" w133 {
          tunnel: [w139 w145] -> w137
          tunnel: w136 -> [w139 w144]
          tunnel: w135 -> [w140 w143]
          tunnel: [w140 w142] -> w134
          frame False {
          }
          frame True {
            n32 = xnode "Read/Write Control"("FPGA VI Reference In"=w143, "error in"=w144, "snapshot"=TRUE) -> ("FPGA VI Reference Out"=w142:refnum<k20>, "error out"=w145:errorcluster)
          }
        }
      }
      frame #1 {
        n33 = flat-sequence {
          tunnel: w160 -> [w169]
          tunnel: w159 -> [w168]
          tunnel: w153 -> [w165]
          tunnel: [w167] -> w163
          tunnel: [w166] -> w162
          tunnel: [w165] -> w161
          tunnel: w150 -> [w164]
          tunnel: [w200] -> w157
          tunnel: w163 -> [w202]
          tunnel: w162 -> [w201]
          tunnel: w161 -> [w199]
          tunnel: [w199] -> w152
          tunnel: [w198] -> w151
          frame #0 {
            n34 = case shown="True" w165 {
              tunnel: w169 -> [w173 w197]
              tunnel: w168 -> [w172 w196]
              tunnel: [w171 w195] -> w166
              tunnel: [w170 w194] -> w167
              tunnel: w164 -> [_ w193]
              frame False {
                n35 = disable-structure shown="Enabled" {
                  disable-tunnel: w173 -> [w180 w183]
                  disable-tunnel: w172 -> [w178 w182]
                  disable-tunnel: [w177 w182] -> w171
                  disable-tunnel: [w174 w183] -> w170
                  frame Disabled {
                    n36 = xnode "Invoke Method"("FPGA VI Reference In"=w180, "error in"=w178, "Number of Elements"=u32 0) -> ("FPGA VI Reference Out"=w176:refnum<k20>, "error out"=w175:errorcluster, "Elements Remaining"=w179:u32)  [unwired: 1 in, 1 out]
                    n37 = xnode "Invoke Method"("FPGA VI Reference In"=w176, "error in"=w175, "Number of Elements"=w179) -> ("FPGA VI Reference Out"=w174:refnum<k20>, "error out"=w177:errorcluster)  [unwired: 1 in, 2 out]
                  }
                  frame Enabled {
                  }
                }
              }
              frame True {
                n38 = Multiply(x=w193, y=u32 1024 ("Number of Elements")) -> (x*y=w187:u32)
                n39 = xnode "Invoke Method"("FPGA VI Reference In"=w197, "error in"=w196, "Number of Elements"=w187, "Timeout (ms)"=-1) -> ("FPGA VI Reference Out"=w190:refnum<k20>, "error out"=w189:errorcluster, "Data"=w192:fxp<+/-,12,12>[])  [unwired: 1 out]
                n40 = To Double Precision Float(number=w192) -> (double precision float=→"N-Signals":dbl[])
                n41 = xnode "Invoke Method"("FPGA VI Reference In"=w190, "error in"=w189, "Number of Elements"=u32 0) -> ("FPGA VI Reference Out"=w194:refnum<k20>, "error out"=w195:errorcluster, "Elements Remaining"=→"Elements Remaining Signal":u32)  [unwired: 1 in, 1 out]
              }
            }
          }
          frame #1 {
            n42 = case shown="False" w199 {
              tunnel: [w204 w207] -> w200
              tunnel: w202 -> [w203 w208]
              tunnel: w201 -> [w204 w206]
              tunnel: [w203 w205] -> w198
              frame False {
              }
              frame True {
                n43 = xnode "Read/Write Control"("FPGA VI Reference In"=w208, "error in"=w206, "snapshot"=FALSE) -> ("FPGA VI Reference Out"=w205:refnum<k20>, "error out"=w207:errorcluster)
              }
            }
          }
        }
        n44 = case shown="True" w156 {
          tunnel: w154 -> [w213 w241]
          tunnel: w155 -> [w212 w242]
          tunnel: [w211 w240] -> w158
          tunnel: w150 -> [_ w228]
          tunnel: w148 -> [w210 w226]
          tunnel: w147 -> [_ w225]
          tunnel: [w210 w223] -> w146
          frame False {
            n45 = disable-structure shown="Enabled" {
              disable-tunnel: w213 -> [w219 _]
              disable-tunnel: w212 -> [w216 w221]
              disable-tunnel: [w215 w221] -> w211
              frame Disabled {
                n46 = xnode "Invoke Method"("FPGA VI Reference In"=w219, "error in"=w216, "Number of Elements"=u32 0) -> ("FPGA VI Reference Out"=w217:refnum<k20>, "error out"=w214:errorcluster, "Elements Remaining"=w218:u32)  [unwired: 1 in, 1 out]
                n47 = xnode "Invoke Method"("FPGA VI Reference In"=w217, "error in"=w214, "Number of Elements"=w218) -> ("error out"=w215:errorcluster)  [unwired: 1 in, 3 out]
              }
              frame Enabled {
              }
            }
          }
          frame True {
            # "256x5"
            # "256x5"
            n48 = Multiply(x=w228, y=u32 1024 ("Number of Elements")) -> (x*y=w232:u32)
            n49 = xnode "Invoke Method"("FPGA VI Reference In"=w241, "error in"=w242, "Number of Elements"=w232, "Timeout (ms)"=-1) -> ("FPGA VI Reference Out"=w236:refnum<k20>, "error out"=w237:errorcluster, "Data"=w239:fxp<+,44,44>[])  [unwired: 1 out]
            n50 = To Double Precision Float(number=w239) -> (double precision float=w238:dbl[])
            n51 = Square Root(x=w238) -> (sqrt(x)=w229:dbl[])
            n52 = xnode "Invoke Method"("FPGA VI Reference In"=w236, "error in"=w237, "Number of Elements"=u32 0) -> ("error out"=w240:errorcluster, "Elements Remaining"=→"Elements Remaining FFT":u32)  [unwired: 1 in, 2 out]
            n53 = call "CleanCompleteFFTArray.vi"("Complete FFT Array"=w229, "FFT Size"=512, "#Signals"=w228) -> ("Second Edge Array"=w227:dbl[], "First Edge Array"=w222:dbl[])  [unwired: 7 in]
            "FALLING First Edge N-FFT" <- w222
            "RISING Second Edge N-FFT" <- w227
            n54 = Build Array (concatenate)(w222, w227) -> (w224:dbl[])
            n55 = RT FIFO Write(0:w226, 1:w224, 3:w225) -> (8:w223:refnum<k33>)  [unwired: 2 in, 3 out]
          }
        }
      }
      frame #2 {
        n56 = case shown="False" w246 {
          tunnel: w245 -> [w250 w254]
          tunnel: [w250 w255] -> w244
          frame False {
          }
          frame True {
            n57 = Decrement(x="tieni premuto per") -> (x-1=w251:i32)
            n58 = Greater Or Equal?(x=w254, y=w251) -> (x >= y?=w253:bool)
            n59 = case shown="True" w253 {
              tunnel: w254 -> [w256 _]
              tunnel: [w257 0] -> w255
              frame False {
                n60 = Increment(x=w256) -> (x+1=w257:i32)
              }
              frame True {
                n61 = local write "Snapshot"(FALSE ("Snapshot")) -> ()
              }
            }
          }
        }
      }
    }
    n62 = node-c288() -> ()  [unwired: 1 in, 1 out]
  }
  n63 = while {
    tunnel: w22 -> [w287]
    tunnel: "first bin" -> [w284]
    tunnel: "last bin" -> [w283]
    tunnel: "Windowing" -> [w282]
    tunnel: "#Signals" -> [w281]
    shift-right: [w279] -> _
    shift-left: w11 -> [w266]
    tunnel: w7 -> [w278]
    tunnel: w15 -> [w277]
    tunnel: w14 -> [w276]
    shift-right: [w274] -> _
    shift-left: 0 ("first bin") -> [w275]
    tunnel: w12 -> [w273]
    shift-right: [w272] -> _
    shift-left: w11 -> [w265]
    shift-right: [w260] -> w4
    shift-left: dbl[] [] -> [w261]
    stop <- w280 stop-if-true
    # "VelocityMoving average"
    # "Distance Moving average"
    n64 = Wait (ms)(milliseconds to wait=u32 10 ("millisecond multiple")) -> ()  [unwired: 1 out]
    n65 = RT FIFO Read(0:w287) -> (9:w285:dbl[], 10:w286:bool)  [unwired: 3 in, 3 out]
    n66 = Array Size(array=w265) -> (size(s)=w271:i32)
    n67 = Array Size(array=w266) -> (size(s)=w267:i32)
    n68 = Greater Or Equal?(x=w271, y="#movesignal 2") -> (x >= y?=w270:bool)
    n69 = Greater Or Equal?(x=w267, y="#movesignal") -> (x >= y?=w268:bool)
    n70 = case shown="True" w270 {
      tunnel: w265 -> [w289 w297]
      tunnel: [w289 w294] -> w263
      frame False {
      }
      frame True {
        n71 = call <vilib>:"Std Deviation and Variance.vi"("X"=w297) -> ("mean"=w290:dbl, "standard deviation"=w292:dbl)  [unwired: 1 in, 1 out]
        "moving mean speed" <- w290
        n72 = Subtract(x=w290, y=w292) -> ()  [unwired: 1 out]
        n73 = Add(x=w290, y=w292) -> ()  [unwired: 1 out]
        n74 = Absolute Value(x=w290) -> (abs(x)=w299:dbl)
        n75 = Build Array(w290) -> (w293:dbl[])
        n76 = Divide(x=w292, y=w299) -> (x/y=→"moving standard deviation rel speed":dbl)
        n77 = Array To Cluster(array=w293) -> (cluster=→"Speed and error":T1)
        n78 = Delete From Array(array=w297, length=1, index=0) -> (array with subset deleted=w294:dbl[])  [unwired: 1 out]
      }
    }
    n79 = case shown="True" w268 {
      tunnel: w266 -> [w301 w307]
      tunnel: [w301 w314] -> w264
      tunnel: w261 -> [w300 w306]
      tunnel: [w300 w304] -> w260
      frame False {
      }
      frame True {
        # "coeff empirico"
        n80 = call <vilib>:"Std Deviation and Variance.vi"("X"=w307) -> ("mean"=w305:dbl, "standard deviation"=w309:dbl)  [unwired: 1 in, 1 out]
        "moving mean" <- w305
        n81 = Absolute Value(x=w305) -> (abs(x)=w316:dbl)
        n82 = Divide(x=w309, y=w316) -> (x/y=→"moving standard deviation rel":dbl)
        n83 = Divide(x=w305, y=2.614797e-07 ("Empirical Distance Costant")) -> (x/y=→"moving freq mean":dbl)
        n84 = case shown="True" "Lin Mes" {
          tunnel: w306 -> [w318 w321]
          tunnel: w305 -> [_ w320]
          tunnel: [w318 w319] -> w304
          frame False {
          }
          frame True {
            n85 = Build Array (concatenate)(w321, w320) -> (w319:dbl[])
          }
        }
        n86 = case shown="False" "Mov mean" {
          tunnel: w307 -> [_ w326]
          tunnel: [dbl[] [] ("appended array") w323] -> w314
          frame False {
            # "Mean"
          }
          frame True {
            # "Mov Mean"
            n87 = Delete From Array(array=w326, length=1, index=0) -> (array with subset deleted=w323:dbl[])  [unwired: 1 out]
          }
        }
        n88 = Build Array(w305, w309) -> (w313:dbl[])
        n89 = Array To Cluster(array=w313) -> (cluster=w312:T1)
        n90 = case shown="True" "Plot" {
          tunnel: w312 -> [_ w317]
          frame False {
          }
          frame True {
            "Distance and error" <- w317
          }
        }
        "Distance ONLINE" <- w307
      }
    }
    n91 = case shown="False" w286 {
      tunnel: w285 -> [w366 _]
      tunnel: w284 -> [w362 _]
      tunnel: w283 -> [w361 _]
      tunnel: w282 -> [w360 _]
      tunnel: w281 -> [w357 _]
      tunnel: [w349 w503] -> w279
      tunnel: w278 -> [w346 _]
      tunnel: w277 -> [w345 _]
      tunnel: w276 -> [w344 _]
      tunnel: w275 -> [w343 w504]
      tunnel: [w331 w504] -> w274
      tunnel: w273 -> [w330 _]
      tunnel: [w329 w502] -> w272
      tunnel: w264 -> [w328 w503]
      tunnel: w263 -> [w327 w502]
      frame False {
        w356 = dbl[] [] ("appended array")
        # "window"
        # "ris"
        # "fall"
        n92 = Array Size(array=w366) -> (size(s)=w364:i32)
        n93 = Divide(x=w364, y=2) -> (x/y=w365:dbl)
        n94 = Split 1D Array(array=w366, index=w365) -> (first subarray=w358:dbl[], second subarray=w359:dbl[])
        n95 = while {
          shift-right: [w434] -> _
          shift-left: w358 -> [w446]
          shift-right: [w435] -> _
          shift-left: w359 -> [w445]
          tunnel: w362 -> [w442]
          tunnel: w361 -> [w441]
          tunnel: w360 -> [w420]
          tunnel: w357 -> [w439]
          shift-right: [w419] -> w355
          shift-left: w356 -> [w417]
          shift-right: [w418] -> w354
          shift-left: w356 -> [w416]
          tunnel: w345 -> [w415] mode=indexing
          tunnel: w344 -> [w414] mode=indexing
          tunnel: [w413] -> w341 mode=indexing
          tunnel: [w412] -> w339 mode=indexing
          tunnel: w330 -> [w411]
          i -> [w436]
          stop <- w440 stop-if-true
          w438 = 256 ("x")
          # "ris"
          # "fall"
          # "max bin detect"
          # "Check amplitude & delta"
          # "Amplitude noise"
          n96 = Increment(x=w436) -> (x+1=w437:i32)
          n97 = Equal?(x=w437, y=w439) -> (x = y?=w440:bool)
          n98 = Split 1D Array(array=w446, index=w438) -> (first subarray=w444:dbl[], second subarray=w434:dbl[])
          n99 = Split 1D Array(array=w445, index=w438) -> (first subarray=w443:dbl[], second subarray=w435:dbl[])
          n100 = call "Max Bin Detection.vi"("FFT Array"=w444, "Init Discard Bins"=w442, "Last Discard Bins"=w441) -> ("Max Bin"=w424:i32, "Prev Max Amp"=w423:dbl, "Max Amp"=w422:dbl, "Succ Max Amp"=w421:dbl)  [unwired: 11 in, 2 out]
          n101 = call "Max Bin Detection.vi"("FFT Array"=w443, "Init Discard Bins"=w442, "Last Discard Bins"=w441) -> ("Max Bin"=w425:i32, "Prev Max Amp"=w428:dbl, "Max Amp"=w426:dbl, "Succ Max Amp"=w427:dbl)  [unwired: 11 in, 2 out]
          n102 = case shown="False" "3 point interpolation algorithm" {
            tunnel: [FALSE ("Check Delta Amp Ok?") w454] -> w430
            tunnel: [FALSE ("Check Delta Amp Ok?") w453] -> w429
            tunnel: w428 -> [_ w452]
            tunnel: w427 -> [_ w451]
            tunnel: w423 -> [_ w450]
            tunnel: w421 -> [_ w449]
            frame False {
            }
            frame True {
              w455 = 10.0 ("Max Difference %")
              # "delta diff%"
              n103 = call "Check Delta Amplitude Extreme bins.vi"("Succ Max Amp"=w449, "Max Difference %"=w455, "Prev Max Amp"=w450) -> ("Check Delta Amp Ok?"=w454:bool)  [unwired: 1 in, 1 out]
              n104 = call "Check Delta Amplitude Extreme bins.vi"("Succ Max Amp"=w451, "Max Difference %"=w455, "Prev Max Amp"=w452) -> ("Check Delta Amp Ok?"=w453:bool)  [unwired: 1 in, 1 out]
            }
          }
          n105 = call "Check Amplitude Bin.vi"("Threshold Amp"=w411, "Max Amp"=w422) -> ("Check Amp Ok?"=w433:bool)  [unwired: 2 in]
          n106 = call "Check Amplitude Bin.vi"("Threshold Amp"=w411, "Max Amp"=w426) -> ("Check Amp Ok?"=w432:bool)  [unwired: 2 in]
          n107 = And(x=w433, y=w432) -> (x .and. y?=w431:bool)
          n108 = case shown="True" w431 {
            tunnel: w430 -> [_ w479]
            tunnel: w429 -> [_ w478]
            tunnel: w428 -> [_ w477]
            tunnel: w427 -> [_ w476]
            tunnel: w426 -> [_ w475]
            tunnel: w425 -> [_ w474]
            tunnel: w424 -> [_ w473]
            tunnel: w423 -> [_ w472]
            tunnel: w422 -> [_ w471]
            tunnel: w421 -> [_ w470]
            tunnel: w420 -> [_ w469]
            tunnel: [w458 w464] -> w419
            tunnel: [w457 w463] -> w418
            tunnel: w417 -> [w458 w468]
            tunnel: w416 -> [w457 w467]
            tunnel: w415 -> [_ w466]
            tunnel: w414 -> [_ w465]
            tunnel: [w456 w460] -> w413
            tunnel: [w456 w459] -> w412
            frame False {
              w456 = 0.0
            }
            frame True {
              # "Bin correction"
              # "Interpolation"
              n109 = case shown="False" w479 {
                tunnel: w473 -> [w495 w501]
                tunnel: w472 -> [w493 w500]
                tunnel: w471 -> [w492 w499]
                tunnel: w470 -> [w491 w498]
                tunnel: [w494 w497] -> w462
                tunnel: w469 -> [w496 _]
                frame False {
                  n110 = call "IFFT Bin interpolation.vi"("Max Bin"=w495, "Max Amp"=w492, "Prev Max Amp"=w493, "Succ Max Amp"=w491, "Windowing"=w496) -> ("Interpolate Bin"=w494:dbl)
                }
                frame True {
                  n111 = call "Barycentric method RT.vi"("Next Amp"=w498, "Max Bin"=w501, "Max Amp"=w499, "Prev Amp"=w500) -> ("Bin"=w497:dbl)  [unwired: 7 in]
                }
              }
              n112 = case shown="False" w478 {
                tunnel: w477 -> [w481 w490]
                tunnel: w476 -> [w480 w489]
                tunnel: w475 -> [w482 w488]
                tunnel: w474 -> [w484 w487]
                tunnel: [w483 w486] -> w461
                tunnel: w469 -> [w485 _]
                frame False {
                  n113 = call "IFFT Bin interpolation.vi"("Max Bin"=w484, "Max Amp"=w482, "Prev Max Amp"=w481, "Succ Max Amp"=w480, "Windowing"=w485) -> ("Interpolate Bin"=w483:dbl)
                }
                frame True {
                  n114 = call "Barycentric method RT.vi"("Next Amp"=w489, "Max Bin"=w487, "Max Amp"=w488, "Prev Amp"=w490) -> ("Bin"=w486:dbl)  [unwired: 7 in]
                }
              }
              n115 = Divide(x=w462, y=w466) -> (x/y=w460:dbl)
              n116 = Divide(x=w461, y=w465) -> (x/y=w459:dbl)
              n117 = Build Array (concatenate)(w467, w459) -> (w463:dbl[])
              n118 = Build Array (concatenate)(w468, w460) -> (w464:dbl[])
            }
          }
        }
        n119 = Array Size(array=w355) -> (size(s)=w352:i32)
        "Fall array size" <- w352
        n120 = Array Size(array=w354) -> (size(s)=→"Rise array size":i32)
        n121 = Array To Cluster(array=w341) -> (cluster=→"5 bin FALL":T1)
        n122 = Array To Cluster(array=w339) -> (cluster=→"5 bin RISE":T1)
        n123 = Greater Than 0?(x=w352) -> (x > 0?=w350:bool)
        n124 = case shown="True" w350 {
          tunnel: w355 -> [_ w408]
          tunnel: w354 -> [_ w407]
          tunnel: w328 -> [w387 w395]
          tunnel: [w387 w394] -> w349
          tunnel: w346 -> [_ w393]
          tunnel: w327 -> [w386 w391]
          tunnel: [w386 w389] -> w329
          frame False {
          }
          frame True {
            w409 = 512.0 ("FFT size")
            # "coeff empirico"
            n125 = call <vilib>:"Std Deviation and Variance.vi"("X"=w408) -> ("mean"=w396:dbl, "standard deviation"=w397:dbl)  [unwired: 1 in, 1 out]
            n126 = call <vilib>:"Std Deviation and Variance.vi"("X"=w407) -> ("mean"=w401:dbl, "standard deviation"=w403:dbl)  [unwired: 1 in, 1 out]
            n127 = Absolute Value(x=w401) -> (abs(x)=w402:dbl)
            n128 = Absolute Value(x=w396) -> (abs(x)=w398:dbl)
            n129 = call "Frequency from bin number RT.vi"("FFT size"=w409, "Bin number"=w396, "Sample Rate (S/s)"=w393) -> ("Detected Frequency (Hz)"=w406:dbl)  [unwired: 8 in]
            "Mean Frequency Falling (Hz)" <- w406
            n130 = Divide(x=w403, y=w402) -> (x/y=→"StdDev Rel 2":dbl)
            n131 = call "Frequency from bin number RT.vi"("FFT size"=w409, "Bin number"=w401, "Sample Rate (S/s)"=w393) -> ("Detected Frequency (Hz)"=w405:dbl)  [unwired: 8 in]
            "Mean Frequency Rising (Hz)" <- w405
            n132 = Divide(x=w397, y=w398) -> (x/y=→"StdDev Rel 1":dbl)
            n133 = call "Distance-Velocity from Freq.vi"("freq_rising"=w405, "Empirical Distance Costant"=2.614797e-07, "freq_falling"=w406) -> ("Distance (m)"=w392:dbl, "Mean Frequency"=→"Mean Frequency":dbl, "Velocity (m/s)"=w390:dbl)  [unwired: 2 in]
            "Distance (m)" <- w392
            "Velocity (m/s)" <- w390
            n134 = Build Array (concatenate)(w391, w390) -> (w389:dbl[])
            n135 = Build Array (concatenate)(w395, w392) -> (w394:dbl[])
          }
        }
        n136 = Increment(x=w343) -> (x+1=w332:i32)
        n137 = Equal?(x=w332, y="#meanBin") -> (x = y?=w342:bool)
        n138 = Not(x=w350) -> (.not. x?=→"Warning":bool)
        n139 = feedback #1(T8 [] ("Real Matrix")) -> (w337:T8)
        n140 = feedback #2(T8 [] ("Real Matrix")) -> (w335:T8)
        n141 = case shown="True" w342 {
          tunnel: w339 -> [w372 _]
          tunnel: w341 -> [w373 _]
          tunnel: [w371 w385] -> w336
          tunnel: [w370 w385] -> w338
          tunnel: w337 -> [w369 w384]
          tunnel: w335 -> [w368 w383]
          tunnel: w332 -> [w367 _]
          tunnel: [w367 0] -> w331
          frame False {
            n142 = Build Array (concatenate)(w369, w373) -> (w370:T8)
            n143 = Build Array (concatenate)(w368, w372) -> (w371:T8)
          }
          frame True {
            w385 = T8 [] ("Real Matrix")
            n144 = call "MatrixMean.vi"("Real Matrix"=w384) -> ("DevStd Assoluta"=w375:dbl[], "Mean"=w374:dbl[])  [unwired: 8 in, 1 out]
            n145 = call "MatrixMean.vi"("Real Matrix"=w383) -> ("DevStd Assoluta"=w378:dbl[], "Mean"=w379:dbl[])  [unwired: 8 in, 1 out]
            n146 = Build Array (concatenate)(w374, w375) -> (w376:dbl[])
            n147 = Build Array (concatenate)(w379, w378) -> (w377:dbl[])
            n148 = Array To Cluster(array=w376) -> (cluster=→"5 bin mean/std FALL":T1)
            n149 = Array To Cluster(array=w377) -> (cluster=→"5 bin mean/std RISE":T1)
          }
        }
        n150 = feedback-in #1(w338) -> ()
        n151 = feedback-in #2(w336) -> ()
      }
      frame True {
      }
    }
    n152 = local read "stop"() -> (w280:bool)
  }
  n153 = node-c288(w40) -> ()  [unwired: 1 out]
  n154 = Merge Errors(w53, w54) -> (w58:errorcluster)
  n155 = flat-sequence {
    tunnel: w58 -> [w512]
    tunnel: w51 -> [w507]
    tunnel: w17 -> [w505]
    frame #0 {
      n156 = xnode "Invoke Method"("FPGA VI Reference In"=w507, "error in"=w512) -> ("FPGA VI Reference Out"=w509:refnum<k20>, "error out"=w508:errorcluster)
      n157 = RT FIFO Delete(0:w505) -> ()  [unwired: 2 in, 1 out]
      n158 = property on="stop" class="Bool (strict)"("Value"=FALSE ("stop")) -> ()  [unwired: 2 in, 2 out]
      n159 = xnode "Invoke Method"("FPGA VI Reference In"=w509, "error in"=w508) -> ("FPGA VI Reference Out"=w510:refnum<k20>, "error out"=w511:errorcluster)
      n160 = xnode "Close FPGA VI Reference"("FPGA VI Reference In"=w510, "error in"=w511) -> ()  [unwired: 1 out]
    }
  }
  n161 = call "Linearize Measure Evaluation.vi"("step (m)"="step (m)", "Distance Array"=w4) -> ("Mean error (m)"=→"Mean error (m)":dbl, "Max peak-peak error (m)"=→"Max peak-peak error (m)":dbl)  [unwired: 6 in, 2 out]
